vi "TouchPanel.RingGui.vi"(8 "disableditems":i32[](array[numeric]), 9 "itemnames":string[](array[string]), 10 "ring in":ext, 11 "Message In":string) -> (1 "Canceled":bool, 2 "ring out":ext)   [LabVIEW 2013]
panel:
  out "Listbox":i32(listbox)
  in  "~Right":bool
  in  "~Left":bool
  out "Message":string
  in  "OKButton":bool caption="OkButton"
  in  "CancelButton":bool
  # "Inputs"
  # "Outputs"
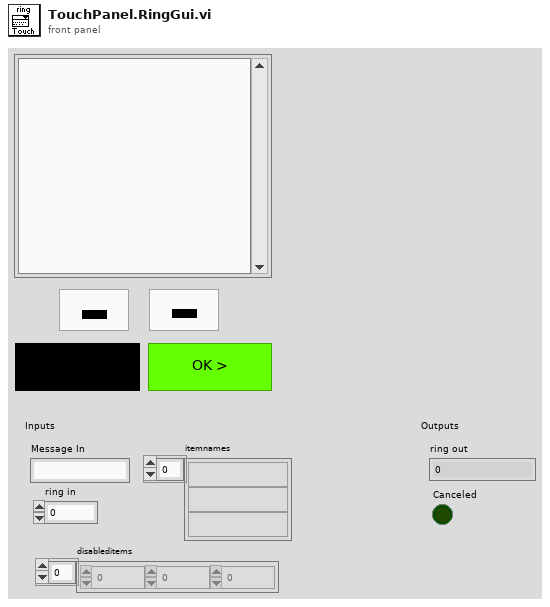
[diagram p1: front panel]
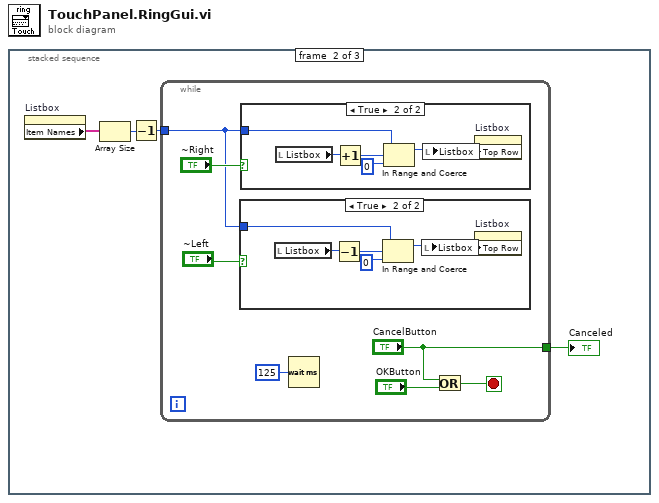
[diagram p0: block diagram]
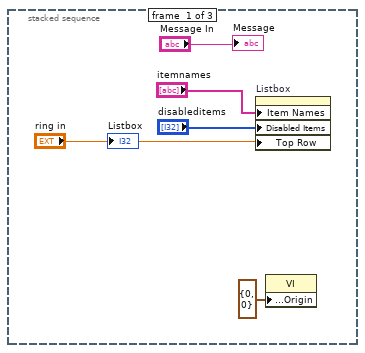
[diagram p2: hidden frame]
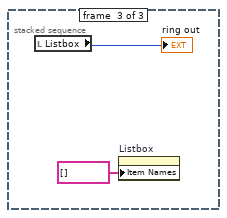
[diagram p5: hidden frame]
diagram:
  n1 = stacked-sequence {
    frame #0 {
      n2 = property on="Listbox" class="LstBox (strict)"("Item Names"="itemnames", "Disabled Items"="disableditems", "Top Row"="ring in") -> ()  [unwired: 2 in, 2 out]
      n3 = property class="VI"("Front Panel Window:Origin"=cluster{"Horizontal":i16, "Vertical":i16} {"Horizontal"=0, "Vertical"=0}) -> ()  [unwired: 2 in, 2 out]
      "Listbox" <- "ring in"
      "Message" <- "Message In"
    }
    frame #1 {
      n4 = property on="Listbox" class="LstBox (strict)"() -> ("Item Names"=w7:string[])  [unwired: 2 in, 2 out]
      n5 = Array Size(array=w7) -> (size(s)=w8:i32)
      n6 = Decrement(x=w8) -> (x-1=w6:i32)
      n7 = while {
        tunnel: ["CancelButton"] -> w9
        tunnel: w6 -> [w10]
        stop <- w15 stop-if-true
        n8 = case shown="True" "~Left" {
          tunnel: w10 -> [_ w18]
          frame False {
          }
          frame True {
            n9 = local read "Listbox"() -> (w21:i32)
            n10 = Decrement(x=w21) -> (x-1=w20:i32)
            n11 = In Range and Coerce(upper limit=w18, x=w20, lower limit=0) -> (coerced(x)=w17:i32)  [unwired: 1 out]
            n12 = local write "Listbox"(w17) -> ()
            n13 = property on="Listbox" class="LstBox (strict)"("Top Row"=w17) -> ()  [unwired: 2 in, 2 out]
          }
        }
        n14 = case shown="True" "~Right" {
          tunnel: w10 -> [_ w23]
          frame False {
          }
          frame True {
            n15 = local read "Listbox"() -> (w26:i32)
            n16 = Increment(x=w26) -> (x+1=w25:i32)
            n17 = In Range and Coerce(upper limit=w23, x=w25, lower limit=0) -> (coerced(x)=w22:i32)  [unwired: 1 out]
            n18 = local write "Listbox"(w22) -> ()
            n19 = property on="Listbox" class="LstBox (strict)"("Top Row"=w22) -> ()  [unwired: 2 in, 2 out]
          }
        }
        n20 = Wait (ms)(milliseconds to wait=u32 125) -> ()  [unwired: 1 out]
        n21 = Or(x="CancelButton", y="OKButton") -> (x .or. y?=w15:bool)
      }
      "Canceled" <- w9
    }
    frame #2 {
      n22 = local read "Listbox"() -> (→"ring out":i32)
      n23 = property on="Listbox" class="LstBox (strict)"("Item Names"=string[] []) -> ()  [unwired: 2 in, 2 out]
    }
  }
